vi "CryptGenRandom.vi"(8 "error in (no error)":errorcluster, 10 "# of bytes (32)":u32=32, 11 "CSP handle in":u32) -> (0 "error out":errorcluster, 1 "random bytes in hex":string, 2 "random bytes array":u8[](array[numeric]), 3 "CSP handle out":u32, 4 "operation status":string)   [LabVIEW 2013]
doc: "Creates cryptographically <b>random bytes</b>.\n\nhttps://msdn.microsoft.com/pl-pl/library/windows/desktop/aa379942(v=vs.85).aspx"
uses:
  advapi32.dll
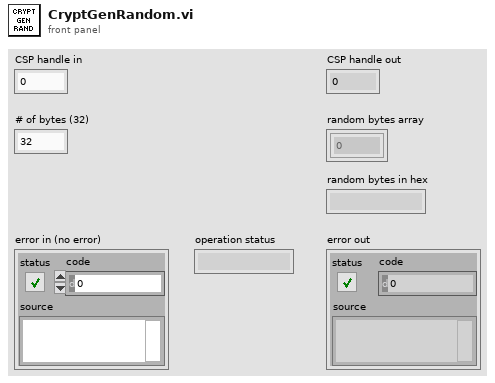
[diagram p1: front panel]
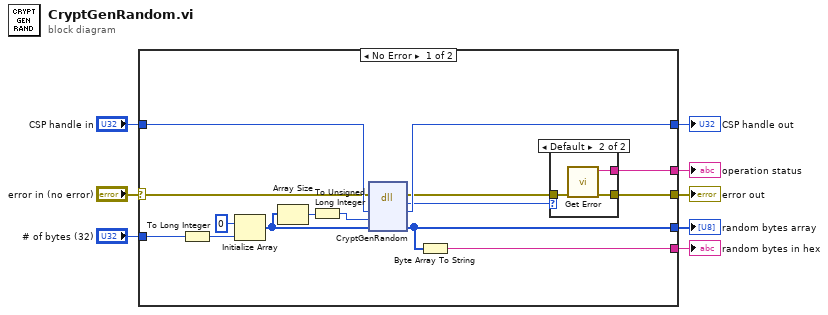
[diagram p0: block diagram]
diagram:
  n1 = case shown="No Error" "error in (no error)" {
    selector: "error in (no error)" -> [w9 w29]
    tunnel: [w21 _] -> w8
    tunnel: [w18 _] -> w7
    tunnel: "CSP handle in" -> [w17 w28]
    tunnel: [w16 w28] -> w5
    tunnel: "# of bytes (32)" -> [w14 _]
    tunnel: [w12 w29] -> w3
    tunnel: [w10 _] -> w2
    frame No Error {
      n2 = To Long Integer(number=w14) -> (32bit integer=w15:i32)
      n3 = Initialize Array(u8 0 ("element"), w15) -> (w20:u8[])
      n4 = Array Size(array=w20) -> (size(s)=w23:i32)
      n5 = To Unsigned Long Integer(number=w23) -> (unsigned 32bit integer=w19:u32)
      n6 = dll-call lib="advapi32.dll" fn="CryptGenRandom"(error in=w9, "hProv"=w17, "dwLen"=w19, "pbBuffer"=w20) -> (error out=w13:errorcluster, "return type"=w11:i32, "hProv"=w16:u32, "pbBuffer"=w18:u8[])  [unwired: 3 in, 1 out]
      n7 = Byte Array To String(unsigned byte array=w18) -> (string=w21:string)
      n8 = case shown="Default" w11 {
        tunnel: w13 -> [w24 w27]
        tunnel: [w24 w26] -> w12
        tunnel: [_ w25] -> w10
        frame 0 {
        }
        frame Default {
          n9 = call "Get Error.vi"("error in (no error)"=w27) -> ("error out"=w26:errorcluster, "lpBuffer"=w25:string)  [unwired: 9 in]
        }
      }
    }
    frame Error {
    }
  }
  "random bytes in hex" <- w8
  "CSP handle out" <- w5
  "random bytes array" <- w7
  "error out" <- w3
  "operation status" <- w2
